vi "Refresh Channel Names and Defaults.vi"(8 "error in (no error)":errorcluster, 10 "engine configuration in":refnum<class "engine configuration.lvclass">, 11 "CVT configuration in":refnum<class "CVT configuration.lvclass">) -> (0 "error out":errorcluster, 2 "engine configuration out":refnum<class "engine configuration.lvclass">, 3 "CVT configuration out":refnum<class "CVT configuration.lvclass">)   [LabVIEW 2013, in "CVT editor node.lvclass"]
uses:
  CVT editor node.lvclass
  <vilib>/NI/Module Execution Interface/Engine Configuration/engine configuration.lvclass
  configuration/CVT configuration.lvclass
  <vilib>/NI/Configuration Framework/serializable configuration/NISE_CEF_serializable configuration.lvclass/NISE_CEF_serializable configuration.ctl
  configuration/CVT configuration.lvclass/CVT configuration.ctl
  <vilib>/NI/Tag Bus/tag/tag descriptor.lvclass/tag descriptor.ctl
  <vilib>/NI/Tag Bus/tag/write tag name.vi
  <vilib>/NI/Tag Bus/tag/read tag name.vi
  <vilib>/NI/Configuration Framework/serializable configuration/Read UID.vi
  configuration/Read channels.vi
  <vilib>/Utility/LVClass/Get LV Class Name.vi
  <vilib>/NI/Configuration Framework/error generator/NISE_error generator.vi
  <vilib>/NI/Tag Bus Module Framework/channel/TBM channel.lvclass
  <vilib>/NI/Tag Bus/tag/tag descriptor.lvclass
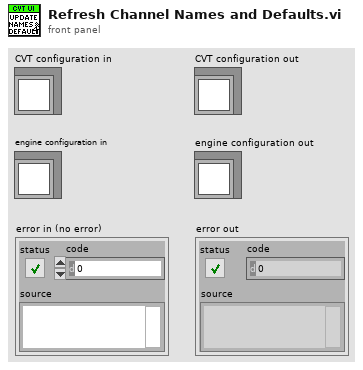
[diagram p1: front panel]
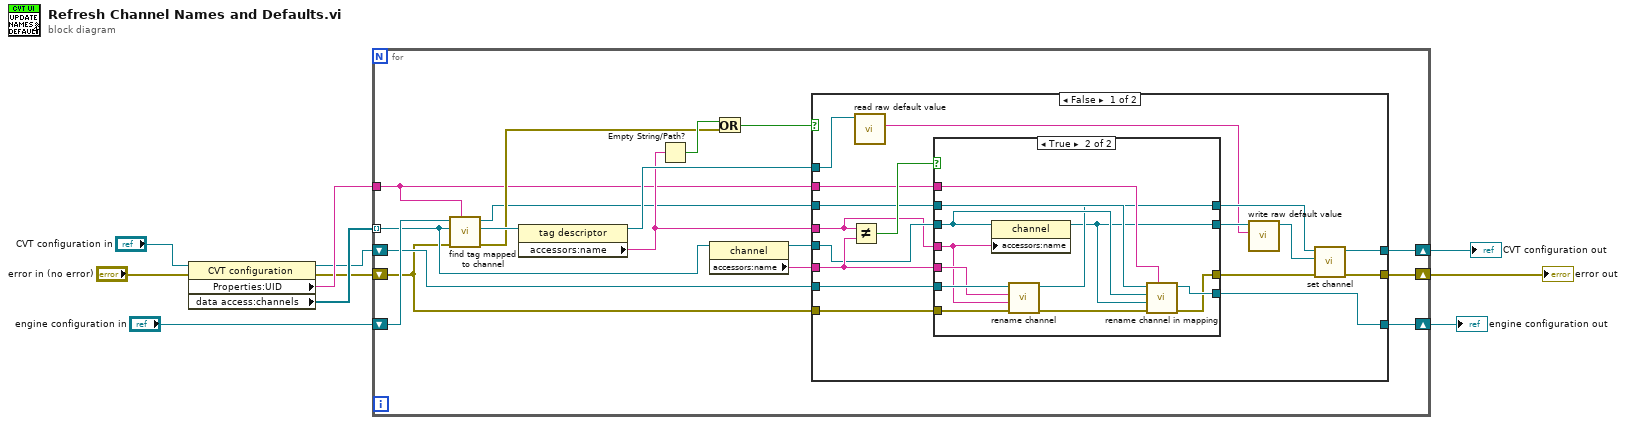
[diagram p0: block diagram]
diagram:
  n1 = property class="CVT configuration"(reference="CVT configuration in", error in="error in (no error)") -> (reference out=w4:refnum<class "CVT configuration.lvclass">, error out=w5:errorcluster, "Properties:UID"=w7:string, "data access:channels"=w8:refnum<class "TBM channel.lvclass">[])
  n2 = for {
    tunnel: w8 -> [w23] mode=indexing
    tunnel: w7 -> [w15]
    shift-right: [w13] -> w1
    shift-left: w5 -> [w14]
    shift-right: [w12] -> w3
    shift-left: w4 -> [w17]
    shift-right: [w11] -> w2
    shift-left: "engine configuration in" -> [w27]
    n3 = call <vilib>:"find tag mapped to channel.vi"("owner"=w15, "error in"=w14, "channel"=w23, "engine configuration in"=w27) -> ("error out"=w24:errorcluster, "tag"=w26:refnum<class "tag descriptor.lvclass">, "engine configuration out"=w16:refnum<class "engine configuration.lvclass">)  [unwired: 5 in]
    n4 = property class="tag descriptor"(reference=w26) -> (reference out=w21:refnum<class "tag descriptor.lvclass">, "accessors:name"=w20:string)  [unwired: 1 in, 1 out]
    n5 = Empty String/Path?(string/path=w20) -> (empty?=w25:bool)
    n6 = property class="channel"(reference=w23) -> (reference out=w18:refnum<class "TBM channel.lvclass">, "accessors:name"=w19:string)  [unwired: 1 in, 1 out]
    n7 = Or(x=w25, y=w24) -> (x .or. y?=w22:bool)
    n8 = case shown="False" w22 {
      tunnel: w21 -> [w29 _]
      tunnel: w20 -> [w40 _]
      tunnel: w19 -> [w42 _]
      tunnel: w18 -> [w41 _]
      tunnel: w17 -> [w43 w62]
      tunnel: w16 -> [w39 w63]
      tunnel: w15 -> [w38 _]
      tunnel: w14 -> [w37 w61]
      tunnel: [w32 w61] -> w13
      tunnel: [w31 w62] -> w12
      tunnel: [w30 w63] -> w11
      frame False {
        n9 = Not Equal?(x=w40, y=w42) -> (x != y?=w44:bool)
        n10 = call <vilib>:"read raw default value.vi"("system tag in"=w29) -> ("raw default"=w28:string)  [unwired: 8 in, 2 out]
        n11 = case shown="True" w44 {
          tunnel: w43 -> [w48 w60]
          tunnel: w42 -> [_ w59]
          tunnel: w41 -> [w46 w55]
          tunnel: w40 -> [_ w58]
          tunnel: w39 -> [w47 w57]
          tunnel: w38 -> [_ w56]
          tunnel: [w48 w53] -> w35
          tunnel: [w47 w52] -> w30
          tunnel: [w45 w51] -> w33
          tunnel: w37 -> [w45 w50]
          tunnel: [w46 w49] -> w36
          frame False {
          }
          frame True {
            n12 = property class="channel"(reference=w55, "accessors:name"=w58) -> (reference out=w49:refnum<class "TBM channel.lvclass">)  [unwired: 1 in, 1 out]
            n13 = call "rename channel.vi"("error in"=w50, "new name"=w58, "old name"=w59, "CVT configuration in"=w60) -> ("error out"=w54:errorcluster, "CVT configuration out"=w53:refnum<class "CVT configuration.lvclass">)  [unwired: 6 in]
            n14 = call <vilib>:"rename channel in mapping.vi"("owner ID"=w56, "error in"=w54, "new channel"=w49, "old channel"=w55, "engine configuration in"=w57) -> ("error out"=w51:errorcluster, "engine configuration out"=w52:refnum<class "engine configuration.lvclass">)  [unwired: 5 in]
          }
        }
        n15 = call <vilib>:"write raw default value.vi"("raw default"=w28, "system tag in"=w36) -> ("system tag out"=w34:refnum<class "TBM channel.lvclass">)  [unwired: 8 in, 1 out]
        n16 = call "set channel.vi"("error in"=w33, "TBM channel in"=w34, "CVT configuration in"=w35) -> ("error out"=w32:errorcluster, "CVT configuration out"=w31:refnum<class "CVT configuration.lvclass">)  [unwired: 7 in]
      }
      frame True {
      }
    }
  }
  "engine configuration out" <- w2
  "CVT configuration out" <- w3
  "error out" <- w1
